vi "ErrorHandling_ErrorQueueSize.vi"(8 "Fehler (Eingang, kein Fehler)":errorcluster caption="Error_In", 11 "Referenz_In":refnum<visa-resource-name>) -> (0 "Fehler (Ausgang)":errorcluster caption="Error_Out", 1 "communication_data":T1, 2 "# of errors":i32, 3 "Referenz_Out":refnum<visa-resource-name>)   [LabVIEW 2018, in "OXYGEN.lvlib"]
doc: "Queries the Error Queue number of elements"
uses:
  OXYGEN.lvlib
  TypeDefs/Cluster_RawCommData.ctl
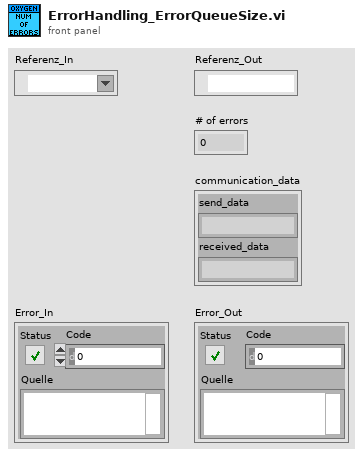
[diagram p1: front panel]
types:
  T1 = typedef "OXYGEN.lvlib/Cluster_RawCommData.ctl" = cluster{"send_data":string, "received_data":string}
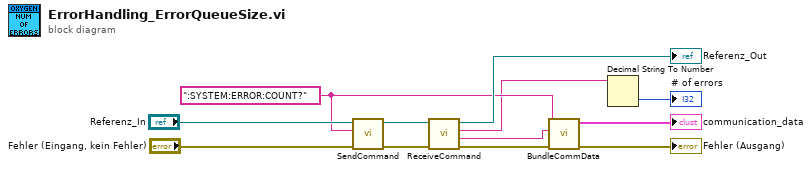
[diagram p0: block diagram]
diagram:
  w6 = ":SYSTEM:ERROR:COUNT?" ("Schreibpuffer")
  n1 = call "SendCommand.vi"("error in (no error)"="Fehler (Eingang, kein Fehler)", "String to Send"=w6, "OXY_SCPI Reseource In"="Referenz_In") -> ("error out"=w8:errorcluster, "OXY_SCPI Reseource Out"=w7:refnum<visa-resource-name>)  [unwired: 7 in]
  n2 = call "ReceiveCommand.vi"("error in (no error)"=w8, "OXY_SCPI Reseource In"=w7) -> ("error out"=w4:errorcluster, "received Data with Header"=w5:string, "received Data"=w2:string, "OXY_SCPI Reseource Out"=→"Referenz_Out":refnum<visa-resource-name>)  [unwired: 6 in]
  n3 = call "BundleCommData.vi"("error in (no error)"=w4, "received_data"=w5, "send_data"=w6) -> ("error out"=→"Fehler (Ausgang)":errorcluster, "communication_data"=→"communication_data":T1)  [unwired: 7 in]
  n4 = Decimal String To Number(string=w2) -> (number=→"# of errors":i32)  [unwired: 2 in, 1 out]
